vi "Scan List.vi"(2 "Add Comma (True)":bool=TRUE, 7 "Scan List (Empty)":string) -> (8 "Scan List Out":string)   [LabVIEW 2015, in "Keithley 27XX.lvlib"]
doc: "The Scan List VI converts a comma separated list of channels into a instrument recognizable scan list."
uses:
  Keithley 27XX.lvlib
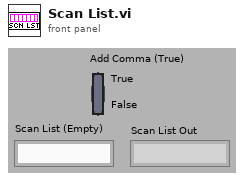
[diagram p1: front panel]
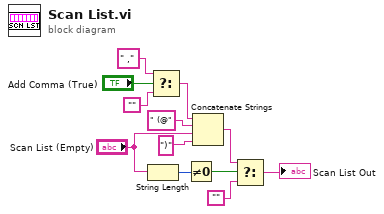
[diagram p0: block diagram]
diagram:
  n1 = String Length(string="Scan List (Empty)") -> (length=w12:i32)
  n2 = Select(t=" ,", s="Add Comma (True)", f="") -> (s? t:f=w1:string)
  n3 = Not Equal To 0?(x=w12) -> (x != 0?=w11:bool)
  n4 = Concatenate Strings(w1, " (@" ("string"), "Scan List (Empty)", ")" ("string")) -> (w8:string)
  n5 = Select(t=w8, s=w11, f="") -> (s? t:f=→"Scan List Out":string)
